vi "CAN refresh.vi"(4 "error in (no error)":errorcluster, 6 "Output image":u8[](array[numeric]), 7 "CANopen in":refnum<class "CANopen.lvclass">) -> (0 "error out":errorcluster, 2 "Changed?":bool, 3 "CANopen out":refnum<class "CANopen.lvclass">)   [LabVIEW 2026, in "canopen_.lvlib" / "CANopen.lvclass"]
doc: "Checks for heartbeat errors with \"Heartbeat check\" and synchronizes the outputs with \"Sync outputs\"."
uses:
  CANopen.lvclass
  CANopen.lvclass/CANopen.ctl
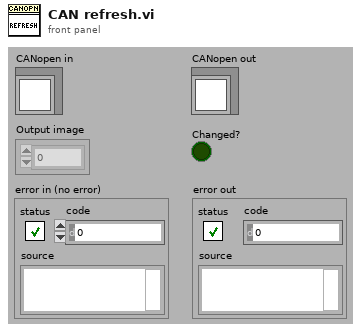
[diagram p1: front panel]
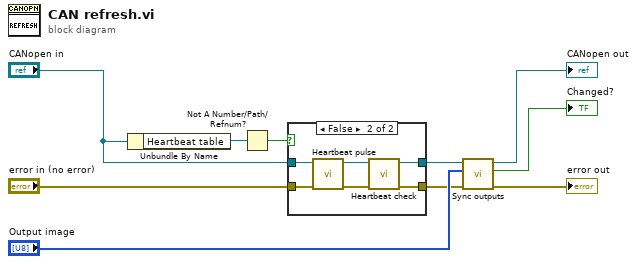
[diagram p0: block diagram]
diagram:
  n1 = Unbundle By Name("CANopen in") -> ("Heartbeat table"=w2:refnum<vi>)
  n2 = Not A Number/Path/Refnum?(number/path/refnum=w2) -> (NaN/Path/Refnum?=w1:bool)
  n3 = case shown="False" w1 {
    tunnel: "error in (no error)" -> [w11 w18]
    tunnel: "CANopen in" -> [w12 w17]
    tunnel: [w11 w14] -> w5
    tunnel: [w12 w13] -> w4
    frame True {
    }
    frame False {
      n4 = call "Heartbeat pulse.vi"("error in"=w18, "CANopen in"=w17) -> ("error out"=w15:errorcluster, "CANopen out"=w16:refnum<class "CANopen.lvclass">)  [unwired: 1 in, 3 out]
      n5 = call "Heartbeat check.vi"("error in"=w15, "CANopen in"=w16) -> ("error out"=w14:errorcluster, "CANopen out"=w13:refnum<class "CANopen.lvclass">)  [unwired: 4 out]
    }
  }
  n6 = call "Sync outputs.vi"("error in (no error)"=w5, "Output image"="Output image", "CANopen in"=w4) -> ("error out"=→"error out":errorcluster, "Changed?"=→"Changed?":bool, "CANopen out"=→"CANopen out":refnum<class "CANopen.lvclass">)  [unwired: 2 out]
